vi "XYZ Print.vi"(0 "VISA resource name":refnum<visa-resource-name>, 5 "XYZ":dbl[](array[numeric]), 7 "Microstep Size (0)":dbl=0.047625, 9 "Speed (mm/s^2)":dbl, 11 "Device and Axis":string[][](array[string])) -> (4 "VISA resource name out":refnum<visa-resource-name>)   [LabVIEW 2018, in "Stage Actor.lvlib" / "Stage.lvclass"]
uses:
  Stage.lvclass
  2b28d5d4-d6db-40e0-90ca-f53d2c79782f.vi
  a669cd2a-0701-48a6-9b34-f17b4ef90bc9.vi
  b1e5870b-3d07-4142-ba0c-87b2a000721a.vi
  <instrlib>/Zaber A Series/Zaber A Series.lvlib
panel:
  in  "error constant":errorcluster
  out "error out":errorcluster
  in  "Units (0: microsteps)":u16(ring)=2 items=["microsteps", "microns", "millimeters", "inches"]
  in  "Movement Type (0: relative)":u16(ring) items=["relative", "absolute"]
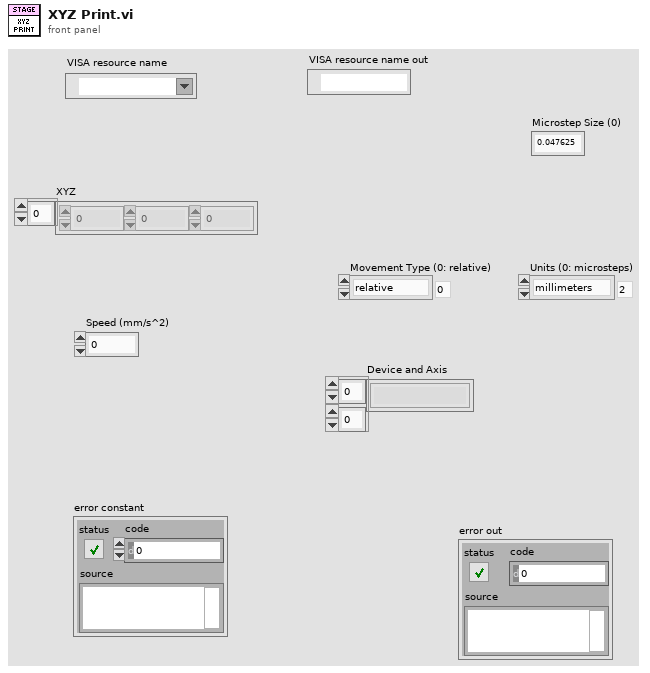
[diagram p1: front panel]
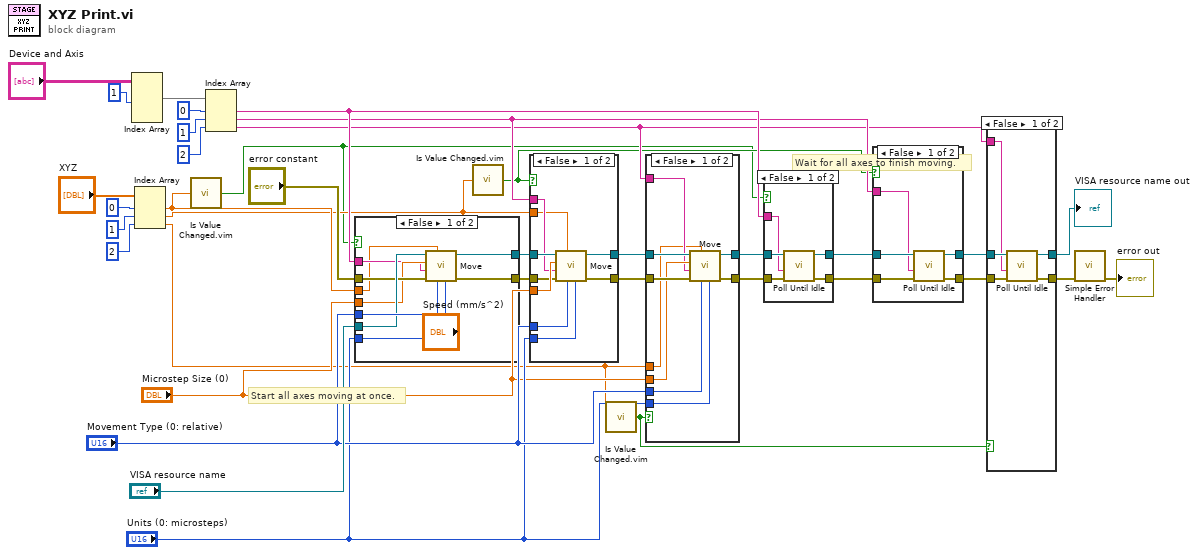
[diagram p0: block diagram]
diagram:
  # "Start all axes moving at once."
  # "Wait for all axes to finish moving."
  n1 = Index Array(array="Device and Axis", index (col) #1=1 ("disabled index (col)")) -> (element #1=w30:string[])  [unwired: 3 in, 1 out]
  n2 = Index Array(array="XYZ", index #1=0 ("index"), index #2=1 ("index"), index #3=2 ("index")) -> (element #1=w6:dbl, element #2=w5:dbl, element #3=w4:dbl)
  n3 = call "Is Value Changed.vim"("value"=w6) -> ("changed or first call?"=w1:bool)
  n4 = Index Array(array=w30, index #1=0 ("index"), index #2=1 ("index"), index #3=2 ("index")) -> (element #1=w25:string, element #2=w24:string, element #3=w23:string)
  n5 = case shown="False" w1 {
    tunnel: "Units (0: microsteps)" -> [w46 _]
    tunnel: [w45 w48] -> w16
    tunnel: "Movement Type (0: relative)" -> [w44 _]
    tunnel: "VISA resource name" -> [w43 w48]
    tunnel: "error constant" -> [w42 w47]
    tunnel: [w41 w47] -> w15
    tunnel: "Microstep Size (0)" -> [w40 _]
    tunnel: w25 -> [w39 _]
    tunnel: w6 -> [w38 _]
    frame False {
      n6 = call <instrlib>:"Move.vi"("Units (0: microsteps)"=w46, "Movement Type (0: relative)"=w44, "Move Distance (0)"=w38, "error in (no error)"=w42, "Device and Axis"=w39, "Microstep Size (0)"=w40, "VISA resource name"=w43) -> ("error out"=w41:errorcluster, "VISA resource name out"=w45:refnum<visa-resource-name>)  [unwired: 3 in]
    }
    frame True {
    }
  }
  n7 = call "Is Value Changed.vim"("value"=w5) -> ("changed or first call?"=w2:bool)
  n8 = case shown="False" w2 {
    tunnel: "Units (0: microsteps)" -> [w57 _]
    tunnel: [w56 w59] -> w14
    tunnel: "Movement Type (0: relative)" -> [w55 _]
    tunnel: w16 -> [w54 w59]
    tunnel: w15 -> [w51 w58]
    tunnel: [w50 w58] -> w13
    tunnel: "Microstep Size (0)" -> [w53 _]
    tunnel: w24 -> [w52 _]
    tunnel: w5 -> [w49 _]
    frame False {
      n9 = call <instrlib>:"Move.vi"("Units (0: microsteps)"=w57, "Movement Type (0: relative)"=w55, "Move Distance (0)"=w49, "error in (no error)"=w51, "Device and Axis"=w52, "Microstep Size (0)"=w53, "VISA resource name"=w54) -> ("error out"=w50:errorcluster, "VISA resource name out"=w56:refnum<visa-resource-name>)  [unwired: 3 in]
    }
    frame True {
    }
  }
  n10 = call "Is Value Changed.vim"("value"=w4) -> ("changed or first call?"=w3:bool)
  n11 = case shown="False" w3 {
    tunnel: "Units (0: microsteps)" -> [w68 _]
    tunnel: [w67 w70] -> w12
    tunnel: "Movement Type (0: relative)" -> [w66 _]
    tunnel: w14 -> [w65 w70]
    tunnel: w13 -> [w64 w69]
    tunnel: [w63 w69] -> w11
    tunnel: "Microstep Size (0)" -> [w62 _]
    tunnel: w23 -> [w61 _]
    tunnel: w4 -> [w60 _]
    frame False {
      n12 = call <instrlib>:"Move.vi"("Units (0: microsteps)"=w68, "Movement Type (0: relative)"=w66, "Move Distance (0)"=w60, "error in (no error)"=w64, "Device and Axis"=w61, "Microstep Size (0)"=w62, "VISA resource name"=w65) -> ("error out"=w63:errorcluster, "VISA resource name out"=w67:refnum<visa-resource-name>)  [unwired: 3 in]
    }
    frame True {
    }
  }
  n13 = case shown="False" w1 {
    tunnel: w12 -> [w75 w77]
    tunnel: w25 -> [w74 _]
    tunnel: w11 -> [w73 w76]
    tunnel: [w72 w76] -> w17
    tunnel: [w71 w77] -> w18
    frame False {
      n14 = call <instrlib>:"Poll Until Idle.vi"("error in (no error)"=w73, "Device and Axis"=w74, "VISA resource name"=w75) -> ("error out"=w72:errorcluster, "VISA resource name out"=w71:refnum<visa-resource-name>)  [unwired: 7 in]
    }
    frame True {
    }
  }
  n15 = case shown="False" w2 {
    tunnel: w18 -> [w82 w84]
    tunnel: w24 -> [w81 _]
    tunnel: w17 -> [w80 w83]
    tunnel: [w79 w83] -> w19
    tunnel: [w78 w84] -> w20
    frame False {
      n16 = call <instrlib>:"Poll Until Idle.vi"("error in (no error)"=w80, "Device and Axis"=w81, "VISA resource name"=w82) -> ("error out"=w79:errorcluster, "VISA resource name out"=w78:refnum<visa-resource-name>)  [unwired: 7 in]
    }
    frame True {
    }
  }
  n17 = case shown="False" w3 {
    tunnel: w20 -> [w89 w91]
    tunnel: w23 -> [w88 _]
    tunnel: w19 -> [w87 w90]
    tunnel: [w86 w90] -> w22
    tunnel: [w85 w91] -> w21
    frame False {
      n18 = call <instrlib>:"Poll Until Idle.vi"("error in (no error)"=w87, "Device and Axis"=w88, "VISA resource name"=w89) -> ("error out"=w86:errorcluster, "VISA resource name out"=w85:refnum<visa-resource-name>)  [unwired: 7 in]
    }
    frame True {
    }
  }
  "VISA resource name out" <- w21
  n19 = call <vilib>:"Simple Error Handler.vi"("error in (no error)"=w22) -> ("error out"=→"error out":errorcluster)  [unwired: 4 in, 4 out]
